vi "Add Block Diagram Content.vi"(8 "error in (no error)":errorcluster, 10 "ModuleLoop":T1, 11 "Wheel Speed Sensor in":refnum<class "Wheel Speed Sensor.lvclass">) -> (0 "error out":errorcluster, 2 "Term Refnum":refnum<vi>, 3 "Wheel Speed Sensor out":refnum<class "Wheel Speed Sensor.lvclass">)   [LabVIEW 2015, in "Wheel Speed Sensor.lvclass"]
uses:
  Wheel Speed Sensor.lvclass
  Loop/Block Diagram/Module.Refs.ctl
  <vilib>/Utility/miscctls.llb/LVPointTypeDef.ctl
  FPGA Addon Output/FPGAAddon.SpecialityOutputs.Generate.Parameters.ctl
  IO Class/Read IP Core Path.vi
  IO Class/Read Signal Name.vi
  FPGA Addon Output/FPGA Addon Output.lvclass
  Loop/Structures/Structures.lvclass
  Loop/Block Diagram/Block Diagram.lvclass
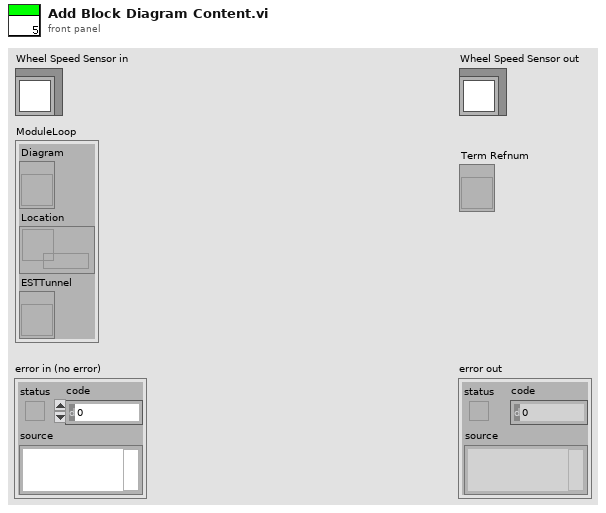
[diagram p1: front panel]
types:
  T1 = typedef "Block Diagram.lvclass/Module.Refs.ctl" = cluster{"Diagram":refnum<vi>, "Location":refnum<data-value>, "ESTTunnel":refnum<vi>}
  T2 = typedef "FPGA Addon Output.lvclass/FPGAAddon.SpecialityOutputs.Generate.Parameters.ctl" = cluster{"Parent":refnum<vi>, "subVI path":path, "location":T3, "IO Name":string}
  T3 = typedef "LVPointTypeDef.ctl" = cluster{"Horizontal":i16, "Vertical":i16}
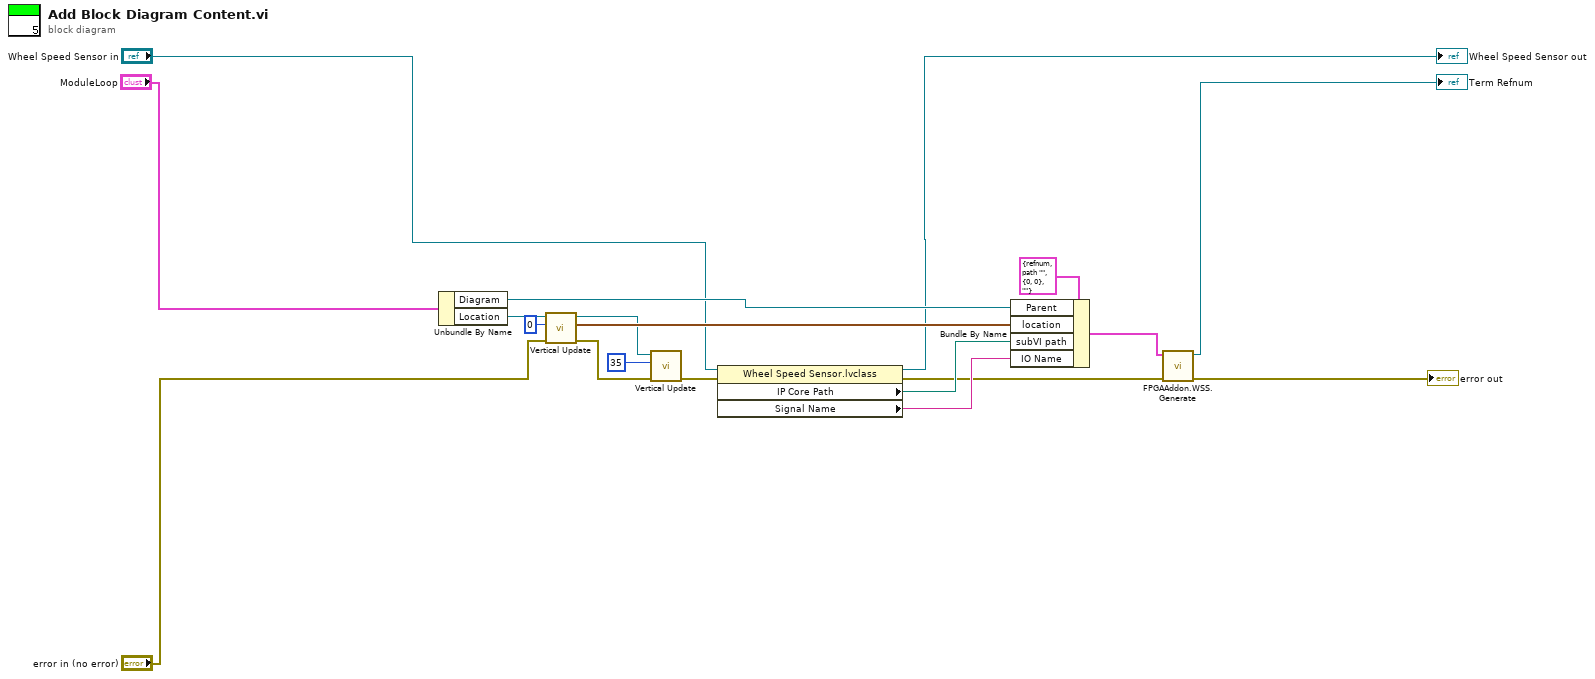
[diagram p0: block diagram]
diagram:
  n1 = Unbundle By Name("ModuleLoop") -> ("Diagram"=w9:refnum<vi>, "Location"=w14:refnum<data-value>)
  n2 = call "Vertical Update.vi"("error in (no error)"="error in (no error)", "Vertical Change"=i16 0, "Location"=w14) -> ("error out"=w11:errorcluster, "location out"=w15:T3, "Location"=w13:refnum<data-value>)  [unwired: 6 in]
  n3 = call "Vertical Update.vi"("error in (no error)"=w11, "Vertical Change"=i16 35, "Location"=w13) -> ("error out"=w10:errorcluster)  [unwired: 6 in, 2 out]
  n4 = property class="Wheel Speed Sensor.lvclass"(reference="Wheel Speed Sensor in", error in=w10) -> (reference out=→"Wheel Speed Sensor out":refnum<class "Wheel Speed Sensor.lvclass">, error out=w4:errorcluster, "IP Core Path"=w18:path, "Signal Name"=w17:string)
  n5 = Bundle By Name(cluster=T2 {"Parent"=refnum, "subVI path"=path "", "location"={"Horizontal"=0, "Vertical"=0}, "IO Name"=""} ("Parameters"), "Parent"=w9, "location"=w15, "subVI path"=w18, "IO Name"=w17) -> (w3:T2)
  n6 = call "FPGAAddon.WSS.Generate.vi"("error in (no error)"=w4, "Parameters"=w3) -> ("error out"=→"error out":errorcluster, "Output.Ref"=→"Term Refnum":refnum<vi>)  [unwired: 8 in]
